vi "Comando_Quick_Silver.vi"(5 "COMANDO COMPLETO":string="COUDE UART1 CHAVEAR OFF") -> (0 "RESP CHAV. 2":string, 1 "RESPOSTA":string, 2 "RESP CHAV. 1":string)   [LabVIEW 2018]
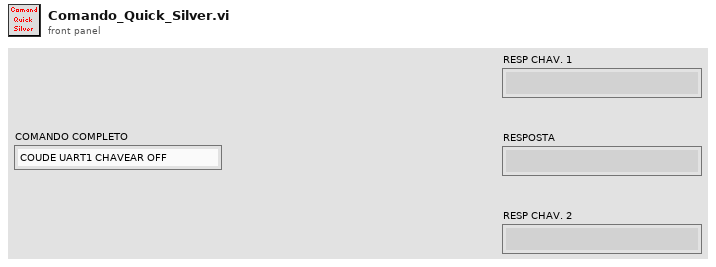
[diagram p1: front panel]
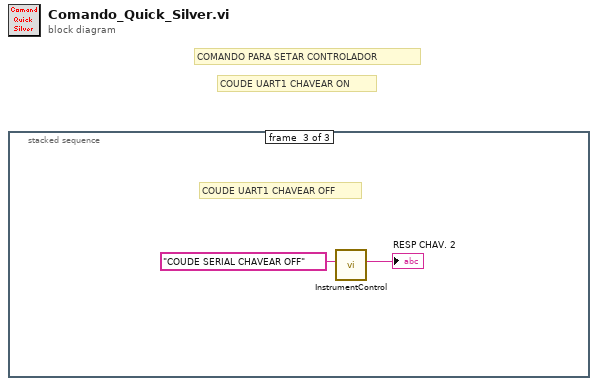
[diagram p0: block diagram]
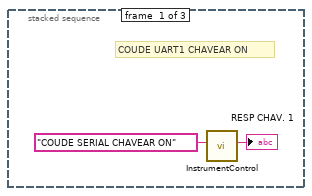
[diagram p2: hidden frame]
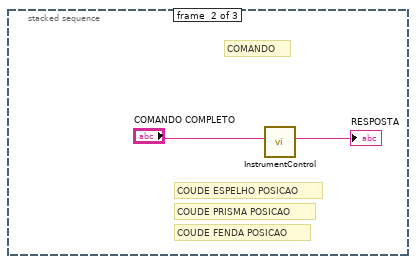
[diagram p3: hidden frame]
diagram:
  # "COUDE UART1 CHAVEAR ON"
  # "COMANDO PARA SETAR CONTROLADOR"
  n1 = stacked-sequence {
    frame #0 {
      # "COUDE UART1 CHAVEAR ON"
      n2 = call "InstrumentControl.vi"("Input Message"="COUDE SERIAL CHAVEAR ON") -> ("Output Message"=→"RESP CHAV. 1":string)  [unwired: 9 in, 1 out]
    }
    frame #1 {
      # "COUDE FENDA POSICAO"
      # "COUDE PRISMA POSICAO"
      # "COUDE ESPELHO POSICAO"
      # "COMANDO"
      n3 = call "InstrumentControl.vi"("Input Message"="COMANDO COMPLETO") -> ("Output Message"=→"RESPOSTA":string)  [unwired: 9 in, 1 out]
    }
    frame #2 {
      # "COUDE UART1 CHAVEAR OFF"
      n4 = call "InstrumentControl.vi"("Input Message"="COUDE SERIAL CHAVEAR OFF") -> ("Output Message"=→"RESP CHAV. 2":string)  [unwired: 9 in, 1 out]
    }
  }
